vi "SECoP-addPropertyBoolean.vi"(8 "error in (no error)":errorcluster, 9 "property value":bool, 10 "property name":string, 11 "DLL path (in)":T1) -> (0 "error out":errorcluster, 3 "DLL path (out)":T1)   [LabVIEW 2023, in "SECoP.lvlib"]
doc: "Call <b>\"SECoP-addPropertyBoolean.vi\"</b> to append a SECoP boolean property to the last SEC node, module, command or parameter. This is a convenience function like \"SECoP-addProperty.vi\" with an boolean true/false value.\n\n<b>DLL path</b> input and output of cluster from \"SECoP-Initialize.vi\"\n<b>property name</b> name of property\n<b>property value</b> value of the property"
uses:
  SECoP.lvlib
  SECoP-libraries.ctl
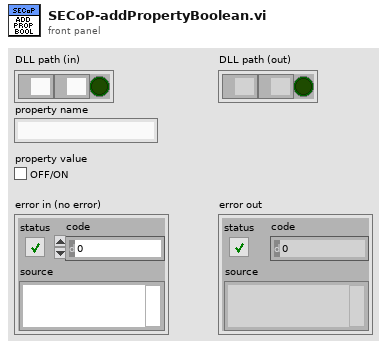
[diagram p1: front panel]
types:
  T1 = typedef "SECoP.lvlib/SECoP-libraries.ctl" = cluster{"serverDLL":path, "variantDLL":path, "cleanup_mode":bool}
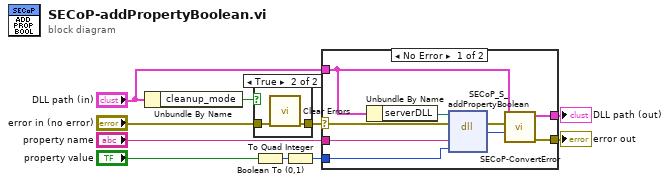
[diagram p0: block diagram]
diagram:
  n1 = Unbundle By Name("DLL path (in)") -> ("cleanup_mode"=w7:bool)
  n2 = case shown="True" w7 {
    tunnel: "error in (no error)" -> [w11 w13]
    tunnel: [w11 w12] -> w5
    frame False {
    }
    frame True {
      n3 = call <vilib>:"Clear Errors.vi"("error in (no error)"=w13) -> ("error out"=w12:errorcluster)  [unwired: 5 in, 1 out]
    }
  }
  n4 = Boolean To (0,1)(Boolean="property value") -> (0, 1=w2:i16)
  n5 = To Quad Integer(1:w2) -> (0:w1:i64)
  n6 = case shown="No Error" w5 {
    selector: w5 -> [w19 w23]
    tunnel: "DLL path (in)" -> [w15 w24]
    tunnel: [w21 w24] -> w10
    tunnel: [w22 w23] -> w9
    tunnel: "property name" -> [w18 _]
    tunnel: w1 -> [w17 _]
    frame No Error {
      n7 = Unbundle By Name(w15) -> ("serverDLL"=w14:path)
      n8 = dll-call lib="Z:/Praktische Aufgaben/SECoP-LabVIEW2015/32bit/SECoP32.dll" fn="SECoP_S_addPropertyBoolean"(path in=w14, error in=w19, "Name"=w18, "Value"=w17) -> (error out=w20:errorcluster, "return type"=w16:i32)  [unwired: 3 in, 1 out]
      n9 = call "SECoP-ConvertError.vi"("return code"=w16, "error in (no error)"=w20, "DLL path (in)"=w15) -> ("error out"=w22:errorcluster, "DLL path (out)"=w21:T1)  [unwired: 7 in]
    }
    frame Error {
    }
  }
  "DLL path (out)" <- w10
  "error out" <- w9
